vi "Read Minor Frames.vi"(8 "error in":errorcluster, 11 "channel ref in":refnum<k20>) -> (0 "error out":errorcluster, 1 "minor frame period (us)":i32, 2 "minor frames":T1[](array[typedef]), 3 "channel ref out":refnum<k20>)   [LabVIEW 2020, in "AIM MIL-STD 1553 Import.lvlib"]
uses:
  AIM MIL-STD 1553 Import.lvlib
  a26b07f3-20e1-4114-9005-43d73faf7b48.vi
  Constants.vi
  Shared/Minor Frame Definition.ctl
  <vilib>/xml/NI_XML.lvlib
  8eca2d5f-955d-43c4-8be7-97fb462d4491.vi
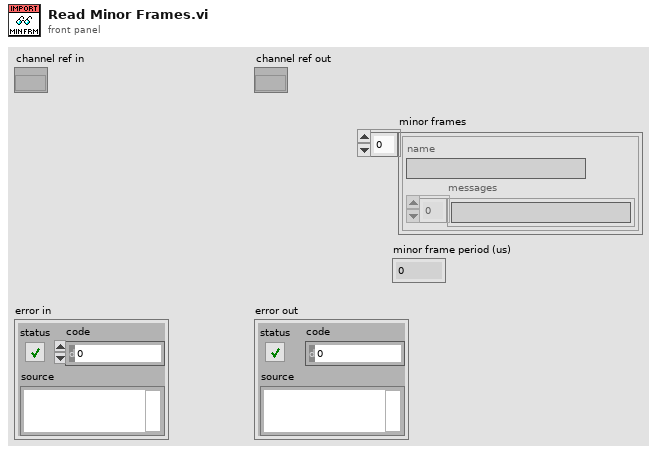
[diagram p1: front panel]
types:
  T1 = typedef "Minor Frame Definition.ctl" = cluster{"name":string, "messages":string[]}
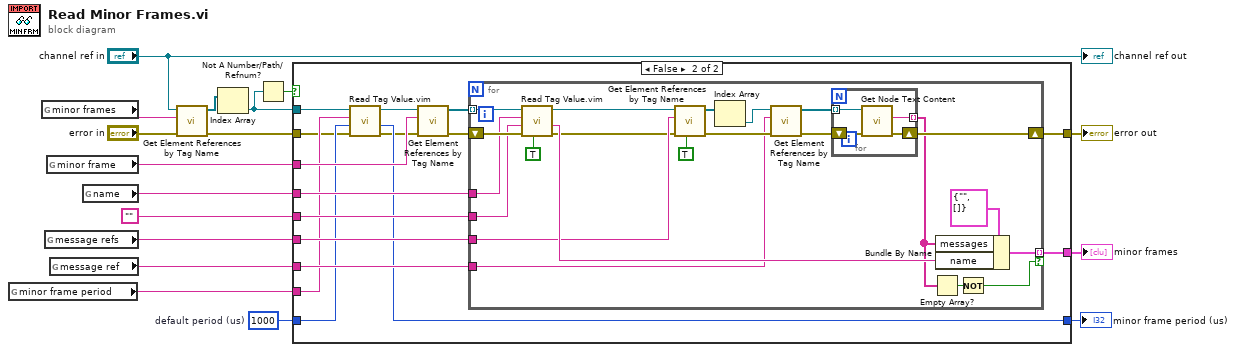
[diagram p0: block diagram]
diagram:
  w1 = 1000  # default period (us)
  n1 = global read "Constants.vi" "minor frame period"() -> (w3:string)
  n2 = global read "Constants.vi" "minor frames"() -> (w8:string)
  n3 = global read "Constants.vi" "message refs"() -> (w5:string)
  n4 = global read "Constants.vi" "minor frame"() -> (w17:string)
  n5 = global read "Constants.vi" "message ref"() -> (w4:string)
  n6 = global read "Constants.vi" "name"() -> (w15:string)
  n7 = call "Get Element References by Tag Name.vi"("error in"="error in", "tag name"=w8, "node in"="channel ref in") -> ("error out"=w10:errorcluster, "array of elements"=w12:refnum<k20>[])  [unwired: 7 in]
  n8 = Index Array(array=w12) -> (element=w9:refnum<k20>)  [unwired: 1 in]
  n9 = Not A Number/Path/Refnum?(number/path/refnum=w9) -> (NaN/Path/Refnum?=w6:bool)
  n10 = case shown="False" w6 {
    tunnel: w17 -> [_ w35]
    tunnel: [w19 w33] -> w16
    tunnel: w15 -> [_ w31]
    tunnel: "" -> [_ w30]
    tunnel: [_ w29] -> w13
    tunnel: w10 -> [w19 w23]
    tunnel: w9 -> [_ w20]
    tunnel: w5 -> [_ w28]
    tunnel: w4 -> [_ w27]
    tunnel: w3 -> [_ w26]
    tunnel: [w18 w25] -> w2
    tunnel: w1 -> [w18 w24]
    frame True {
    }
    frame False {
      n11 = call "Read Tag Value.vim"("error in"=w23, "default"=w24, "tag name"=w26, "node in"=w20) -> ("error out"=w22:errorcluster, "value"=w25:i32, "node out"=w21:refnum<k20>)  [unwired: 5 in]
      n12 = call "Get Element References by Tag Name.vi"("error in"=w22, "tag name"=w35, "node in"=w21) -> ("error out"=w32:errorcluster, "array of elements"=w34:refnum<k20>[])  [unwired: 7 in]
      n13 = for {
        shift-right: [w41] -> w33
        shift-left: w32 -> [w57]
        tunnel: w34 -> [w56] mode=indexing
        tunnel: w31 -> [w55]
        tunnel: w30 -> [w54]
        tunnel: [w51] -> w29 mode=indexing if=w36
        tunnel: w28 -> [w48]
        tunnel: w27 -> [w44]
        n14 = call "Read Tag Value.vim"("required (F)"=TRUE, "error in"=w57, "default"=w54, "tag name"=w55, "node in"=w56) -> ("error out"=w40:errorcluster, "value"=w52:string, "node out"=w39:refnum<k20>)  [unwired: 4 in]
        n15 = call "Get Element References by Tag Name.vi"("required (F)"=TRUE, "error in"=w40, "tag name"=w48, "node in"=w39) -> ("error out"=w45:errorcluster, "array of elements"=w47:refnum<k20>[])  [unwired: 6 in]
        n16 = Index Array(array=w47) -> (element=w46:refnum<k20>)  [unwired: 1 in]
        n17 = call "Get Element References by Tag Name.vi"("error in"=w45, "tag name"=w44, "node in"=w46) -> ("error out"=w42:errorcluster, "array of elements"=w43:refnum<k20>[])  [unwired: 7 in]
        n18 = for {
          tunnel: w43 -> [w61] mode=indexing
          shift-right: [w59] -> w41
          shift-left: w42 -> [w60]
          tunnel: [w58] -> w38 mode=indexing
          n19 = call <vilib>:"Get Node Text Content.vi"("error in (no error)"=w60, "node in"=w61) -> ("error out"=w59:errorcluster, "node text"=w58:string)  [unwired: 7 in, 1 out]
        }
        n20 = Empty Array?(array=w38) -> (empty?=w37:bool)
        n21 = Bundle By Name(cluster=T1 {"name"="", "messages"=[]} ("minor frame definition"), "messages"=w38, "name"=w52) -> (w51:T1)
        n22 = Not(x=w37) -> (.not. x?=w36:bool)
      }
    }
  }
  "error out" <- w16
  "minor frames" <- w13
  "minor frame period (us)" <- w2
  "channel ref out" <- "channel ref in"
